vi "CRYCurve A & B.vi"(7 "X-axis Combination":u16, 8 "Work in":u16(slide), 9 "Curve B":T1={"Name"="", "Curve"=[], "X data"=1, "Y data"=1, "Z data"=1, "X axis"=0, "Y axis"=1, "Z axis"=1, "X unit"="Hz", "Y unit"="", "Z unit"="deg.", "X dB ref"=1.0, "Y dB ref"=1.0, "Z dB ref"=1.0, "single val"=FALSE, "protected"=FALSE, "display X"=TRUE, "display Y"=TRUE, "display Z"=TRUE, "Test Info"="", "Step No."=0, "Plot Settings"={"Color"=0, "Interpolation"=0, "Point Style"=0, "Line Style"=0, "Point Color"=0, "Line Width"=0, "Bar Plot Style"=0, "Fill To"=0}, "AutoProtect"=FALSE} {"Z data" items=["dB", "Lin"]; "X data" items=["dB", "Lin"]; "Y data" items=["dB", "Lin"]; "Z dB ref" format="%.1f"; "Z axis" items=["Log", "Lin"]; "X dB ref" format="%.1f"; "X axis" items=["Log", "Lin"]; "Y axis" items=["Log", "Lin"]; "Y dB ref" format="%.1f"; "Curve"."z" format="%.2f"; "Curve"."y" format="%.2f"; "Curve"."x" format="%.2f"}, 10 "Operator":u16(ring) items=["+", "--", "x", "/"], 11 "Curve A":T1={"Name"="", "Curve"=[], "X data"=1, "Y data"=1, "Z data"=1, "X axis"=0, "Y axis"=1, "Z axis"=1, "X unit"="Hz", "Y unit"="", "Z unit"="deg.", "X dB ref"=1.0, "Y dB ref"=1.0, "Z dB ref"=1.0, "single val"=FALSE, "protected"=FALSE, "display X"=TRUE, "display Y"=TRUE, "display Z"=TRUE, "Test Info"="", "Step No."=0, "Plot Settings"={"Color"=0, "Interpolation"=0, "Point Style"=0, "Line Style"=0, "Point Color"=0, "Line Width"=0, "Bar Plot Style"=0, "Fill To"=0}, "AutoProtect"=FALSE} {"Z data" items=["dB", "Lin"]; "X data" items=["dB", "Lin"]; "Y data" items=["dB", "Lin"]; "Z dB ref" format="%.1f"; "Z axis" items=["Log", "Lin"]; "X dB ref" format="%.1f"; "X axis" items=["Log", "Lin"]; "Y axis" items=["Log", "Lin"]; "Y dB ref" format="%.1f"; "Curve"."z" format="%.2f"; "Curve"."y" format="%.2f"; "Curve"."x" format="%.2f"}) -> (3 "Result":T1={"Name"="", "Curve"=[], "X data"=1, "Y data"=1, "Z data"=1, "X axis"=0, "Y axis"=1, "Z axis"=1, "X unit"="Hz", "Y unit"="", "Z unit"="deg.", "X dB ref"=1.0, "Y dB ref"=1.0, "Z dB ref"=1.0, "single val"=FALSE, "protected"=FALSE, "display X"=TRUE, "display Y"=TRUE, "display Z"=TRUE, "Test Info"="", "Step No."=0, "Plot Settings"={"Color"=0, "Interpolation"=0, "Point Style"=0, "Line Style"=0, "Point Color"=0, "Line Width"=0, "Bar Plot Style"=0, "Fill To"=0}, "AutoProtect"=FALSE} {"Z data" items=["dB", "Lin"]; "X data" items=["dB", "Lin"]; "Y data" items=["dB", "Lin"]; "Z dB ref" format="%.1f"; "Z axis" items=["Log", "Lin"]; "X dB ref" format="%.1f"; "X axis" items=["Log", "Lin"]; "Y axis" items=["Log", "Lin"]; "Y dB ref" format="%.1f"; "Curve"."z" format="%.2f"; "Curve"."y" format="%.2f"; "Curve"."x" format="%.2f"})   [LabVIEW 2013]
doc: "OVERVIEW:\n Sub-vi to perform generalized mathematical operations on arrays which may be different sizes or have different sampling rates, etc."
uses:
  Typedef Control/CRYData Cluster.ctl
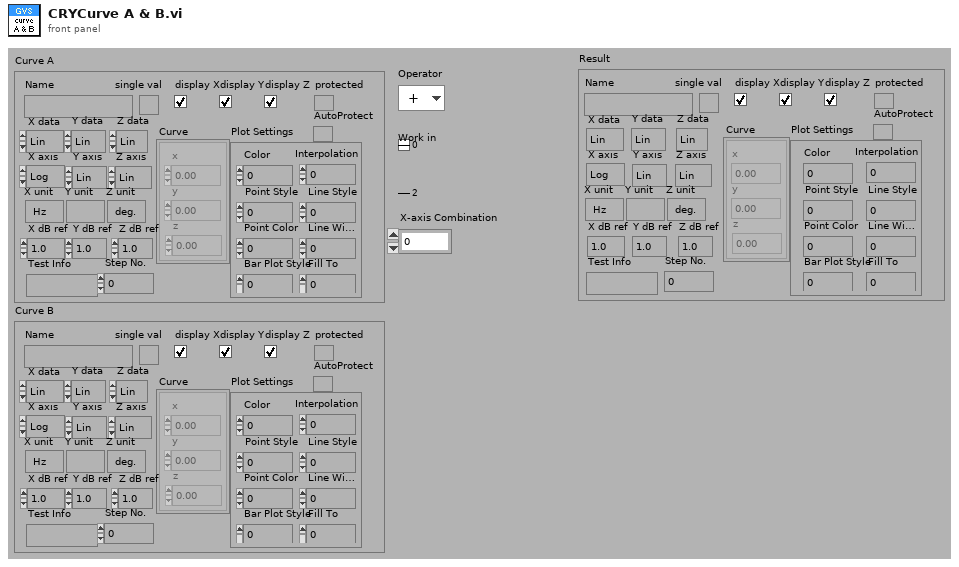
[diagram p1: front panel]
types:
  T1 = typedef "CRYData Cluster.ctl" = cluster{"Name":string, "Curve":cluster{"x":dbl, "y":dbl, "z":dbl}[], "X data":u16, "Y data":u16, "Z data":u16, "X axis":u16, "Y axis":u16, "Z axis":u16, "X unit":string, "Y unit":string, "Z unit":string, "X dB ref":dbl, "Y dB ref":dbl, "Z dB ref":dbl, "single val":bool, "protected":bool, "display X":bool, "display Y":bool, "display Z":bool, "Test Info":string, "Step No.":i32, "Plot Settings":cluster{"Color":u32, "Interpolation":u8, "Point Style":u8, "Line Style":u8, "Point Color":u32, "Line Width":u8, "Bar Plot Style":u8, "Fill To":i16}, "AutoProtect":bool}
  T2 = cluster{"Numeric":dbl, "Y value":dbl, "Y value":dbl}
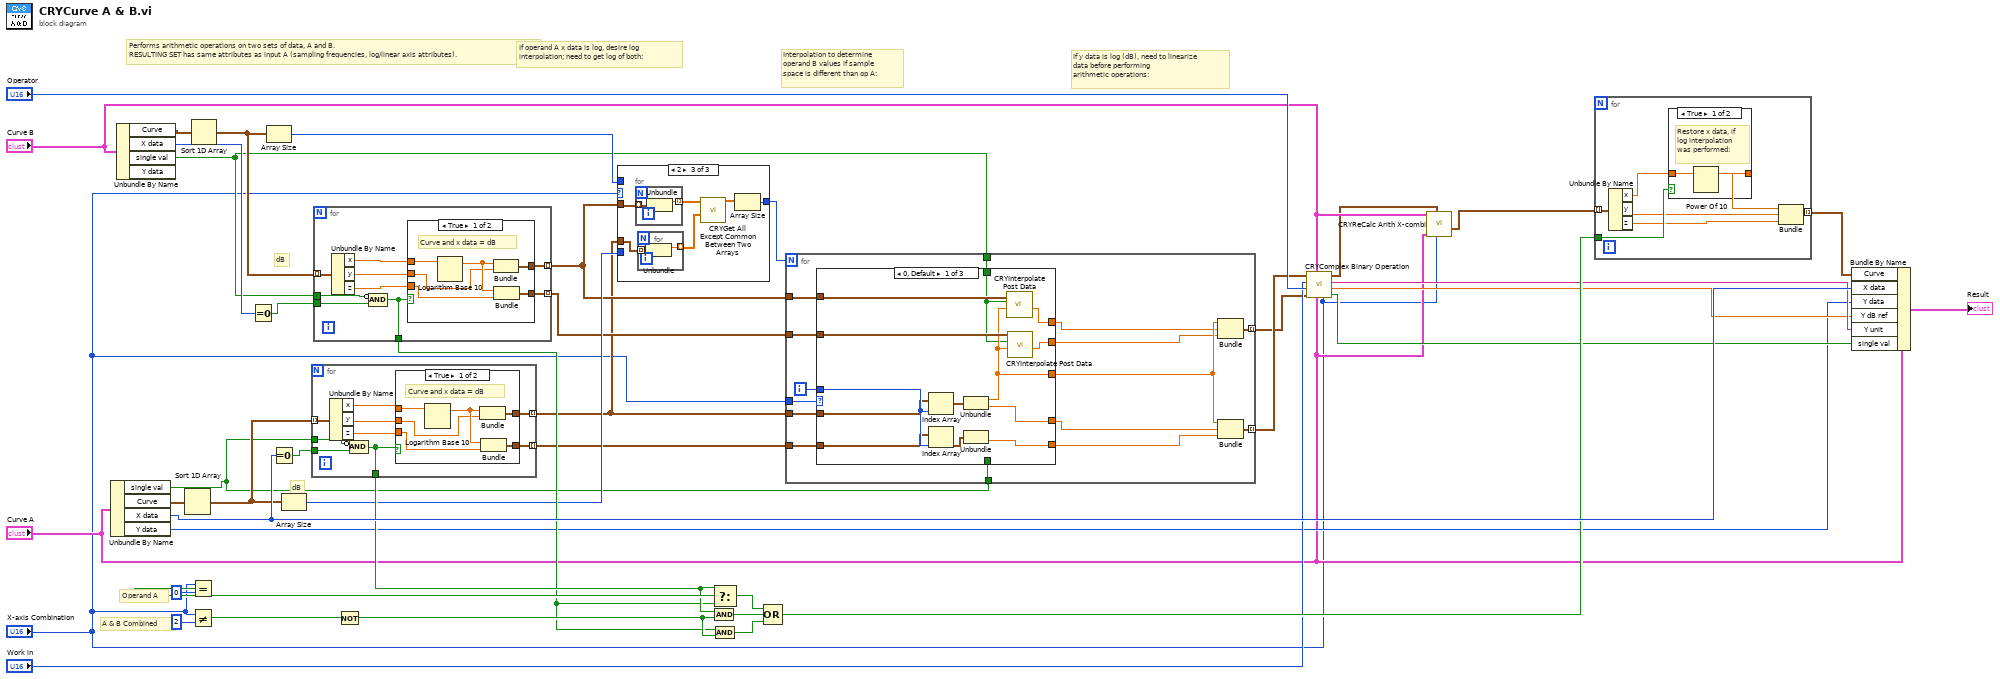
[diagram p0: block diagram]
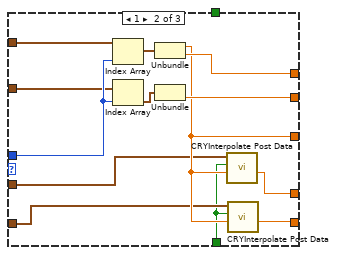
[diagram p2: hidden frame]
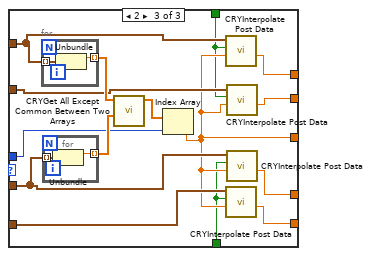
[diagram p3: hidden frame]
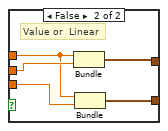
[diagram p6: hidden frame]
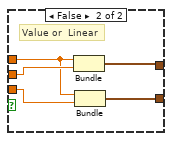
[diagram p8: hidden frame]
diagram:
  # "A & B Combined"
  # "dB"
  # "dB"
  # "Operand A"
  # "If y data is log (dB), need to linearize\ndata before performing \narithmetic operations:"
  # "Interpolation to determine\noperand B values if sample\nspace is different than op A:"
  # "If operand A x data is log, desire log\ninterpolation; need to get log of both:"
  # "Performs arithmetic operations on two sets of data, A and B.\nRESULTING SET has same attributes as input A (sampling frequencies, log/linear axis attributes)."
  n1 = Unbundle By Name("Curve A") -> ("single val"=w6:bool, "Curve"=w26:cluster{"x":dbl, "y":dbl, "z":dbl}[], "X data"=w38:u16, "Y data"=w8:u16)
  n2 = Unbundle By Name("Curve B") -> ("Curve"=w27:cluster{"x":dbl, "y":dbl, "z":dbl}[], "X data"=w41:u16, "single val"=w7:bool)  [unwired: 1 out]
  n3 = Sort 1D Array(array=w26) -> (sorted array=w23:cluster{"x":dbl, "y":dbl, "z":dbl}[])
  n4 = Equal?(x="X-axis Combination", y=u16 0) -> (x = y?=w37:bool)
  n5 = Not Equal?(x="X-axis Combination", y=u16 2) -> (x != y?=w36:bool)
  n6 = Sort 1D Array(array=w27) -> (sorted array=w24:cluster{"x":dbl, "y":dbl, "z":dbl}[])
  n7 = Equal To 0?(x=w41) -> (x = 0?=w43:bool)
  n8 = Array Size(array=w24) -> (size(s)=w22:i32)
  n9 = Equal To 0?(x=w38) -> (x = 0?=w42:bool)
  n10 = Array Size(array=w23) -> (size(s)=w21:i32)
  n11 = for {
    tunnel: w23 -> [w52] mode=indexing
    tunnel: w42 -> [w51]
    tunnel: [w50] -> w34
    tunnel: [w48] -> w17 mode=indexing
    tunnel: [w47] -> w16 mode=indexing
    tunnel: w6 -> [w46]
    n12 = Unbundle By Name(w52) -> ("x"=w45:dbl, "y"=w44:dbl, "z"=w49:dbl)
    n13 = Compound Arithmetic op=AND(invert w46, w51) -> (w50:bool)
    n14 = case shown="True" w50 {
      tunnel: w45 -> [w58 w62]
      tunnel: w44 -> [w56 w63]
      tunnel: w49 -> [w55 w61]
      tunnel: [w54 w60] -> w48
      tunnel: [w53 w59] -> w47
      frame True {
        # "Curve and x data = dB"
        n15 = Logarithm Base 10(1:w58) -> (0:w57:dbl)
        n16 = Bundle(w57, "y"=w56) -> (w54:cluster{dbl, "y":dbl})  [unwired: 1 out]
        n17 = Bundle(w57, "z"=w55) -> (w53:cluster{dbl, "z":dbl})  [unwired: 1 out]
      }
      frame False {
        # "Value or  Linear"
        n18 = Bundle("x"=w62, "y"=w63) -> (w60:cluster{"x":dbl, "y":dbl})  [unwired: 1 out]
        n19 = Bundle("x"=w62, "z"=w61) -> (w59:cluster{"x":dbl, "z":dbl})  [unwired: 1 out]
      }
    }
  }
  n20 = for {
    tunnel: w24 -> [w72] mode=indexing
    tunnel: w43 -> [w68]
    tunnel: [w70] -> w19 mode=indexing
    tunnel: [w69] -> w18 mode=indexing
    tunnel: [w67] -> w33
    tunnel: w7 -> [w66]
    n21 = Unbundle By Name(w72) -> ("x"=w65:dbl, "y"=w64:dbl, "z"=w71:dbl)
    n22 = Compound Arithmetic op=AND(invert w66, w68) -> (w67:bool)
    n23 = case shown="True" w67 {
      tunnel: w65 -> [w78 w82]
      tunnel: w64 -> [w76 w83]
      tunnel: w71 -> [w75 w81]
      tunnel: [w74 w80] -> w70
      tunnel: [w73 w79] -> w69
      frame True {
        # "Curve and x data = dB"
        n24 = Logarithm Base 10(1:w78) -> (0:w77:dbl)
        n25 = Bundle(w77, "y"=w76) -> (w74:cluster{dbl, "y":dbl})  [unwired: 1 out]
        n26 = Bundle(w77, "z"=w75) -> (w73:cluster{dbl, "z":dbl})  [unwired: 1 out]
      }
      frame False {
        # "Value or  Linear"
        n27 = Bundle("x"=w82, "y"=w83) -> (w80:cluster{"x":dbl, "y":dbl})  [unwired: 1 out]
        n28 = Bundle("x"=w82, "z"=w81) -> (w79:cluster{"x":dbl, "z":dbl})  [unwired: 1 out]
      }
    }
  }
  n29 = Not(x=w36) -> (.not. x?=w35:bool)
  n30 = case shown="2" "X-axis Combination" {
    tunnel: w17 -> [_ _ w90]
    tunnel: w19 -> [_ _ w91]
    tunnel: [w84 w85 w87] -> w20
    tunnel: w22 -> [_ w85 _]
    tunnel: w21 -> [w84 _ _]
    frame 0, Default {
    }
    frame 1 {
    }
    frame 2 {
      n31 = for {
        tunnel: w91 -> [w95] mode=indexing
        tunnel: [w94] -> w89 mode=indexing
        n32 = Unbundle(w95) -> ("x"=w94:dbl)  [unwired: 1 out]
      }
      n33 = for {
        tunnel: w90 -> [w93] mode=indexing
        tunnel: [w92] -> w88 mode=indexing
        n34 = Unbundle(w93) -> ("x"=w92:dbl)  [unwired: 1 out]
      }
      n35 = call "CRYGet All Except Common Between Two Arrays.vi"("B"=w88, "A"=w89) -> ("Result"=w86:dbl[])  [unwired: 9 out]
      n36 = Array Size(array=w86) -> (size(s)=w87:i32)
    }
  }
  n37 = And(x=w34, y=w35) -> (x .and. y?=w31:bool)
  n38 = Select(t=w34, s=w37, f=w33) -> (s? t:f=w32:bool)
  n39 = And(x=w33, y=w35) -> (x .and. y?=w30:bool)
  n40 = Compound Arithmetic op=OR(w32, w31, w30) -> (w29:bool)
  n41 = for {
    N: w20 -> [_]
    tunnel: "X-axis Combination" -> [w110]
    tunnel: w19 -> [w108]
    tunnel: w18 -> [w107]
    tunnel: w17 -> [w106]
    tunnel: w16 -> [w105]
    tunnel: [w102] -> w9 mode=indexing
    tunnel: [w101] -> w10 mode=indexing
    tunnel: w7 -> [w99]
    tunnel: w6 -> [w98]
    i -> [w109]
    n42 = case shown="0, Default" w110 {
      tunnel: [w112 w131 w143] -> w97
      tunnel: [w118 w128 w140] -> w96
      tunnel: [w117 w127 w141] -> w103
      tunnel: [w114 w129 w139] -> w104
      tunnel: [w111 w130 w142] -> w100
      tunnel: w108 -> [w116 w132 w147]
      tunnel: w107 -> [w115 w133 w146]
      tunnel: w109 -> [w123 w134 w148]
      tunnel: w106 -> [w122 w126 w145]
      tunnel: w105 -> [w121 w125 w144]
      tunnel: w99 -> [w113 _ w138]
      tunnel: w98 -> [_ w124 w137]
      frame 0, Default {
        n43 = Index Array(array=w122, index=w123) -> (element=w120:cluster{"x":dbl, "y":dbl})
        n44 = Index Array(array=w121, index=w123) -> (element=w119:cluster{"x":dbl, "z":dbl})
        n45 = Unbundle(w120) -> ("x"=w114:dbl, "y"=w118:dbl)
        n46 = Unbundle(w119) -> ("z"=w117:dbl)  [unwired: 1 out]
        n47 = call "CRYInterpolate Post Data.vi"("X value"=w114, "Single Value"=w113, "Curve in"=w116) -> ("Y value"=w112:dbl)  [unwired: 8 in]
        n48 = call "CRYInterpolate Post Data.vi"("X value"=w114, "Single Value"=w113, "Curve in"=w115) -> ("Y value"=w111:dbl)  [unwired: 8 in]
      }
      frame 1 {
        n49 = Index Array(array=w132, index=w134) -> (element=w136:cluster{"x":dbl, "y":dbl})
        n50 = Index Array(array=w133, index=w134) -> (element=w135:cluster{"x":dbl, "z":dbl})
        n51 = Unbundle(w136) -> ("x"=w129:dbl, "y"=w131:dbl)
        n52 = Unbundle(w135) -> ("z"=w130:dbl)  [unwired: 1 out]
        n53 = call "CRYInterpolate Post Data.vi"("X value"=w129, "Single Value"=w124, "Curve in"=w126) -> ("Y value"=w128:dbl)  [unwired: 8 in]
        n54 = call "CRYInterpolate Post Data.vi"("X value"=w129, "Single Value"=w124, "Curve in"=w125) -> ("Y value"=w127:dbl)  [unwired: 8 in]
      }
      frame 2 {
        n55 = for {
          tunnel: w147 -> [w155] mode=indexing
          tunnel: [w154] -> w151 mode=indexing
          n56 = Unbundle(w155) -> ("x"=w154:dbl)  [unwired: 1 out]
        }
        n57 = for {
          tunnel: w145 -> [w153] mode=indexing
          tunnel: [w152] -> w150 mode=indexing
          n58 = Unbundle(w153) -> ("x"=w152:dbl)  [unwired: 1 out]
        }
        n59 = call "CRYGet All Except Common Between Two Arrays.vi"("B"=w150, "A"=w151) -> ("Result"=w149:dbl[])  [unwired: 9 out]
        n60 = Index Array(array=w149, index=w148) -> (element=w139:dbl)
        n61 = call "CRYInterpolate Post Data.vi"("X value"=w139, "Single Value"=w138, "Curve in"=w147) -> ("Y value"=w143:dbl)  [unwired: 8 in]
        n62 = call "CRYInterpolate Post Data.vi"("X value"=w139, "Single Value"=w137, "Curve in"=w144) -> ("Y value"=w141:dbl)  [unwired: 8 in]
        n63 = call "CRYInterpolate Post Data.vi"("X value"=w139, "Single Value"=w138, "Curve in"=w146) -> ("Y value"=w142:dbl)  [unwired: 8 in]
        n64 = call "CRYInterpolate Post Data.vi"("X value"=w139, "Single Value"=w137, "Curve in"=w145) -> ("Y value"=w140:dbl)  [unwired: 8 in]
      }
    }
    n65 = Bundle("Numeric"=w104, "Y value"=w97, "Y value"=w100) -> (w102:T2)  [unwired: 1 in]
    n66 = Bundle("Numeric"=w104, "Y value"=w96, "Y value"=w103) -> (w101:T2)  [unwired: 1 in]
  }
  n67 = call "CRYComplex Binary Operation.vi"("Axis Mode"="X-axis Combination", "A data for units"="Curve A", "B data for units"="Curve B", "Curve B"=w9, "operator"="Operator", "Work in"="Work in", "Curve A"=w10) -> ("Single val out"=w11:bool, "Result dB ref"=w15:dbl, "Result Y unit"=w28:string, "Result"=w3:cluster{"x":dbl, "y":dbl, "z":dbl}[])  [unwired: 1 out]
  n68 = call "CRYReCalc Arith X-combi.vi"("X-axis Combination"="X-axis Combination", "Curve_In"=w3, "Curve A"="Curve A", "Curve B"="Curve B") -> ("Curve_Out"=w1:cluster{"x":dbl, "y":dbl, "z":dbl}[])  [unwired: 7 in]
  n69 = for {
    tunnel: w1 -> [w161] mode=indexing
    tunnel: w29 -> [w162]
    tunnel: [w158] -> w25 mode=indexing
    n70 = Unbundle By Name(w161) -> ("x"=w160:dbl, "y"=w156:dbl, "z"=w159:dbl)
    n71 = case shown="True" w162 {
      tunnel: w160 -> [w164 w165]
      tunnel: [w163 w165] -> w157
      frame True {
        # "Restore x data, if\nlog interpolation\nwas performed:"
        n72 = Power Of 10(x=w164) -> (10^x=w163:dbl)
      }
      frame False {
      }
    }
    n73 = Bundle("x"=w157, "y"=w156, "z"=w159) -> (w158:cluster{"x":dbl, "y":dbl, "z":dbl})  [unwired: 1 out]
  }
  n74 = Bundle By Name(cluster="Curve A", "Curve"=w25, "X data"=w38, "Y data"=w8, "Y dB ref"=w15, "Y unit"=w28, "single val"=w11) -> (→"Result":T1)
